vi "FT_Create_Device_Info_List.vi"() -> (0 "Number of Devices":u32, 1 "FT_Status":u32)   [LabVIEW 2010]
uses:
  FTD2XX.dll
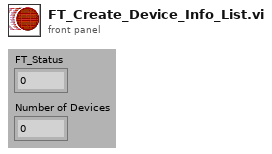
[diagram p1: front panel]
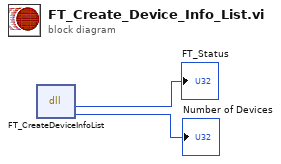
[diagram p0: block diagram]
diagram:
  n1 = dll-call lib="D:/WORK/LabView/#Avesta/D2XX_Functions_7.0/FTD2XX.dll" fn="FT_CreateDeviceInfoList"() -> ("FT_Status"=→"FT_Status":u32, "Number of Devices"=→"Number of Devices":u32)  [unwired: 3 in, 3 out]
